vi "calcDemandedSteps.vi"(8 "error in (no error)":errorcluster, 11 "Model in":refnum<class "Model.lvclass">) -> (0 "error out":errorcluster, 3 "Model out":refnum<class "Model.lvclass">)   [LabVIEW 2013, in "Model.lvclass"]
uses:
  Model.lvclass
  Model.lvclass/Model.ctl
  ApplicationElements/StepperMotor/StepperMotor.lvclass/StepperMotor.ctl
  <userlib>/Common/Component/Application/Application/Application.lvclass/Application.ctl
  ApplicationElements/SystemController/SystemController.lvclass
  ApplicationElements/StepperMotor/StepperMotor.lvclass
  <userlib>/Common/Component/Application/Application/Application.lvclass
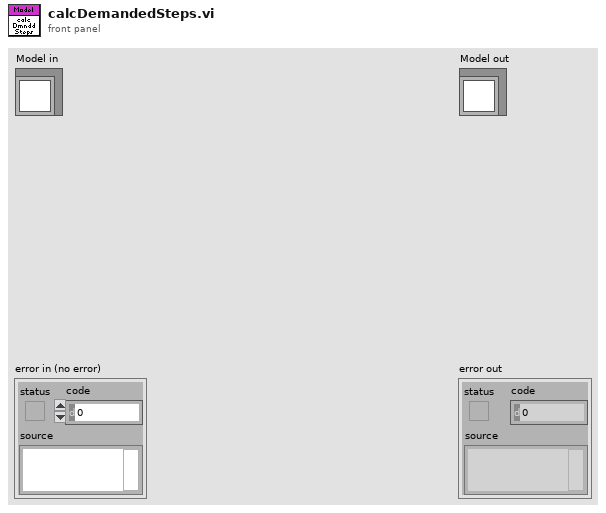
[diagram p1: front panel]
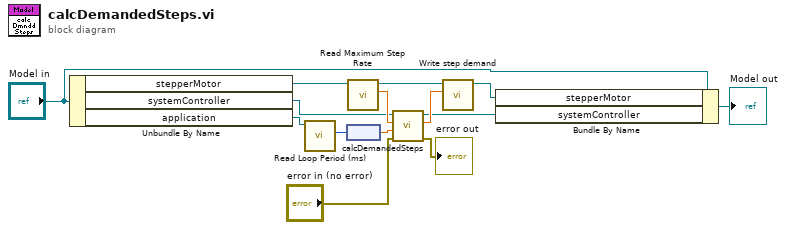
[diagram p0: block diagram]
diagram:
  n1 = Unbundle By Name("Model in") -> ("stepperMotor"=w13:refnum<class "StepperMotor.lvclass">, "systemController"=w5:refnum<class "SystemController.lvclass">, "application"=w3:refnum<class "Application.lvclass">)
  n2 = call <userlib>:"Read Loop Period (ms).vi"("Application in"=w3) -> ("Loop Period (ms)"=w2:u16)  [unwired: 9 in, 1 out]
  n3 = node(w2) -> (w1:dbl[unit])
  n4 = call "Read Maximum Step Rate.vi"("StepperMotor in"=w13) -> ("Maximum Step Rate"=w14:dbl[unit], "StepperMotor out"=w12:refnum<class "StepperMotor.lvclass">)  [unwired: 9 in]
  n5 = call "calcDemandedSteps.vi"("error in (no error)"="error in (no error)", "loopPeriod"=w1, "step rate limit (mag)"=w14, "SystemController in"=w5) -> ("error out"=→"error out":errorcluster, "step demand"=w8:dbl, "SystemController out"=w4:refnum<class "SystemController.lvclass">)  [unwired: 5 in]
  n6 = call "Write step demand.vi"("step demand"=w8, "StepperMotor in"=w12) -> ("StepperMotor out"=w9:refnum<class "StepperMotor.lvclass">)  [unwired: 9 in]
  n7 = Bundle By Name(cluster="Model in", "stepperMotor"=w9, "systemController"=w4) -> (→"Model out":refnum<class "Model.lvclass">)
